vi "File IO - Create Data Folder_SubVIs-某型振动实验台测试系统.vi"(8 "error in":errorcluster, 11 "path input":path) -> (0 "error out":errorcluster, 3 "path output":path)   [LabVIEW 2015]
doc: "判断Data File文件夹是否存在。\n若不存在则创建该文件夹；\n若存在，则传出文件夹路径。"
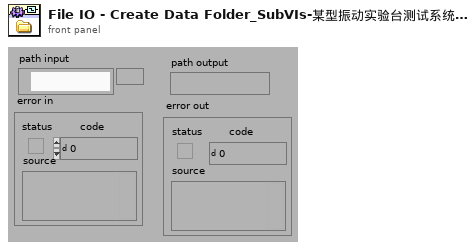
[diagram p1: front panel]
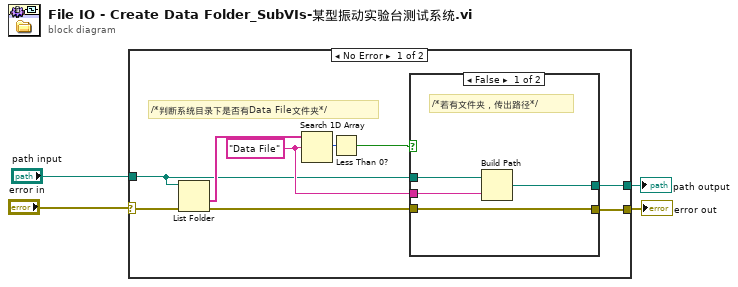
[diagram p0: block diagram]
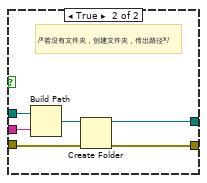
[diagram p2: hidden frame]
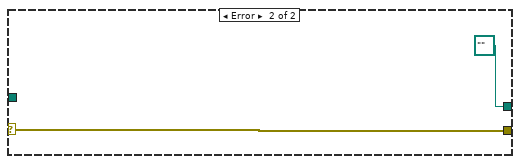
[diagram p3: hidden frame]
diagram:
  n1 = case shown="No Error" "error in" {
    selector: "error in" -> [w7 w25]
    tunnel: [w6 w25] -> w3
    tunnel: "path input" -> [w8 _]
    tunnel: [w5 path "" ("appended path")] -> w1
    frame No Error {
      w12 = "Data File" ("名称或相对路径")
      # "/*判断系统目录下是否有Data File文件夹*/"
      n2 = List Folder(path=w8, error in=w7) -> (folder names=w9:string[], error out=w13:errorcluster)  [unwired: 4 out]
      n3 = Search 1D Array(1D array=w9, element=w12) -> (index of element=w10:i32)  [unwired: 1 out]
      n4 = Less Than 0?(x=w10) -> (x < 0?=w11:bool)
      n5 = case shown="False" w11 {
        tunnel: w8 -> [w16 w23]
        tunnel: w12 -> [w15 w22]
        tunnel: [w14 w18] -> w5
        tunnel: w13 -> [w17 w20]
        tunnel: [w17 w19] -> w6
        frame False {
          # "/*若有文件夹，传出路径*/"
          n6 = Build Path(base path=w16, name or relative path=w15) -> (appended path=w14:path)
        }
        frame True {
          # "/*若没有文件夹，创建文件夹，传出路径*/"
          n7 = Build Path(base path=w23, name or relative path=w22) -> (appended path=w21:path)
          n8 = Create Folder(path (use dialog)=w21, error in=w20) -> (created path=w18:path, error out=w19:errorcluster)  [unwired: 2 out]
        }
      }
    }
    frame Error {
    }
  }
  "error out" <- w3
  "path output" <- w1
